vi "constroi_atp_bakcup.vi"() -> ()   [LabVIEW 2014]
uses:
  <vilib>/Utility/file.llb/Read From Spreadsheet File (DBL).vi
  <vilib>/Utility/file.llb/Read From Spreadsheet File (string).vi
panel:
  in  "Capacitors":string="  N0083A                      1.  .001  36.8                                   0\n  N0083B                      1.  .001  36.8                                   0\n  N0083C                      1.  .001  36.8                                   0\n  N0088A                      1.  .001   9.2                                   0\n  N0090B                      1.  .001   9.2                                   0\n  N0092C                      1.  .001   9.2                                   0"
  out "Switches":string
  out "chaves":dbl[][](array[numeric])
  out "Loads":string
  in  "Frequência (Hz)":dbl=50.0
  in  "Fonte (V)":dbl=4160.0
  out "subarray":dbl[][](array[numeric])
  out "nós":dbl[](array[numeric])
  out "all rows 2":dbl[][](array[numeric]) format="%0.3f"
  out "Linhas":string
  out "Reatances":dbl[][](array[numeric])
  out "Resistances":dbl[][](array[numeric])
  out "config":dbl[](array[numeric])
  out "Para":dbl[](array[numeric])
  out "De":dbl[](array[numeric])
  out "all rows":dbl[][](array[numeric]) format="%0.3f"
  out "Distance (miles)":dbl[](array[numeric])
  out "size(s)":i32[](array[numeric])
  in  "file path (use dialog)":path=path "C:/Users/Flavio/Documents/ATPdata/work/teste.atp"
  out "concatenated string":string
  # "A                B              C"
  # "A"
  # "B"
  # "C"
  # "R     +     X"
  # "R     +     X"
  # "R     +     X"
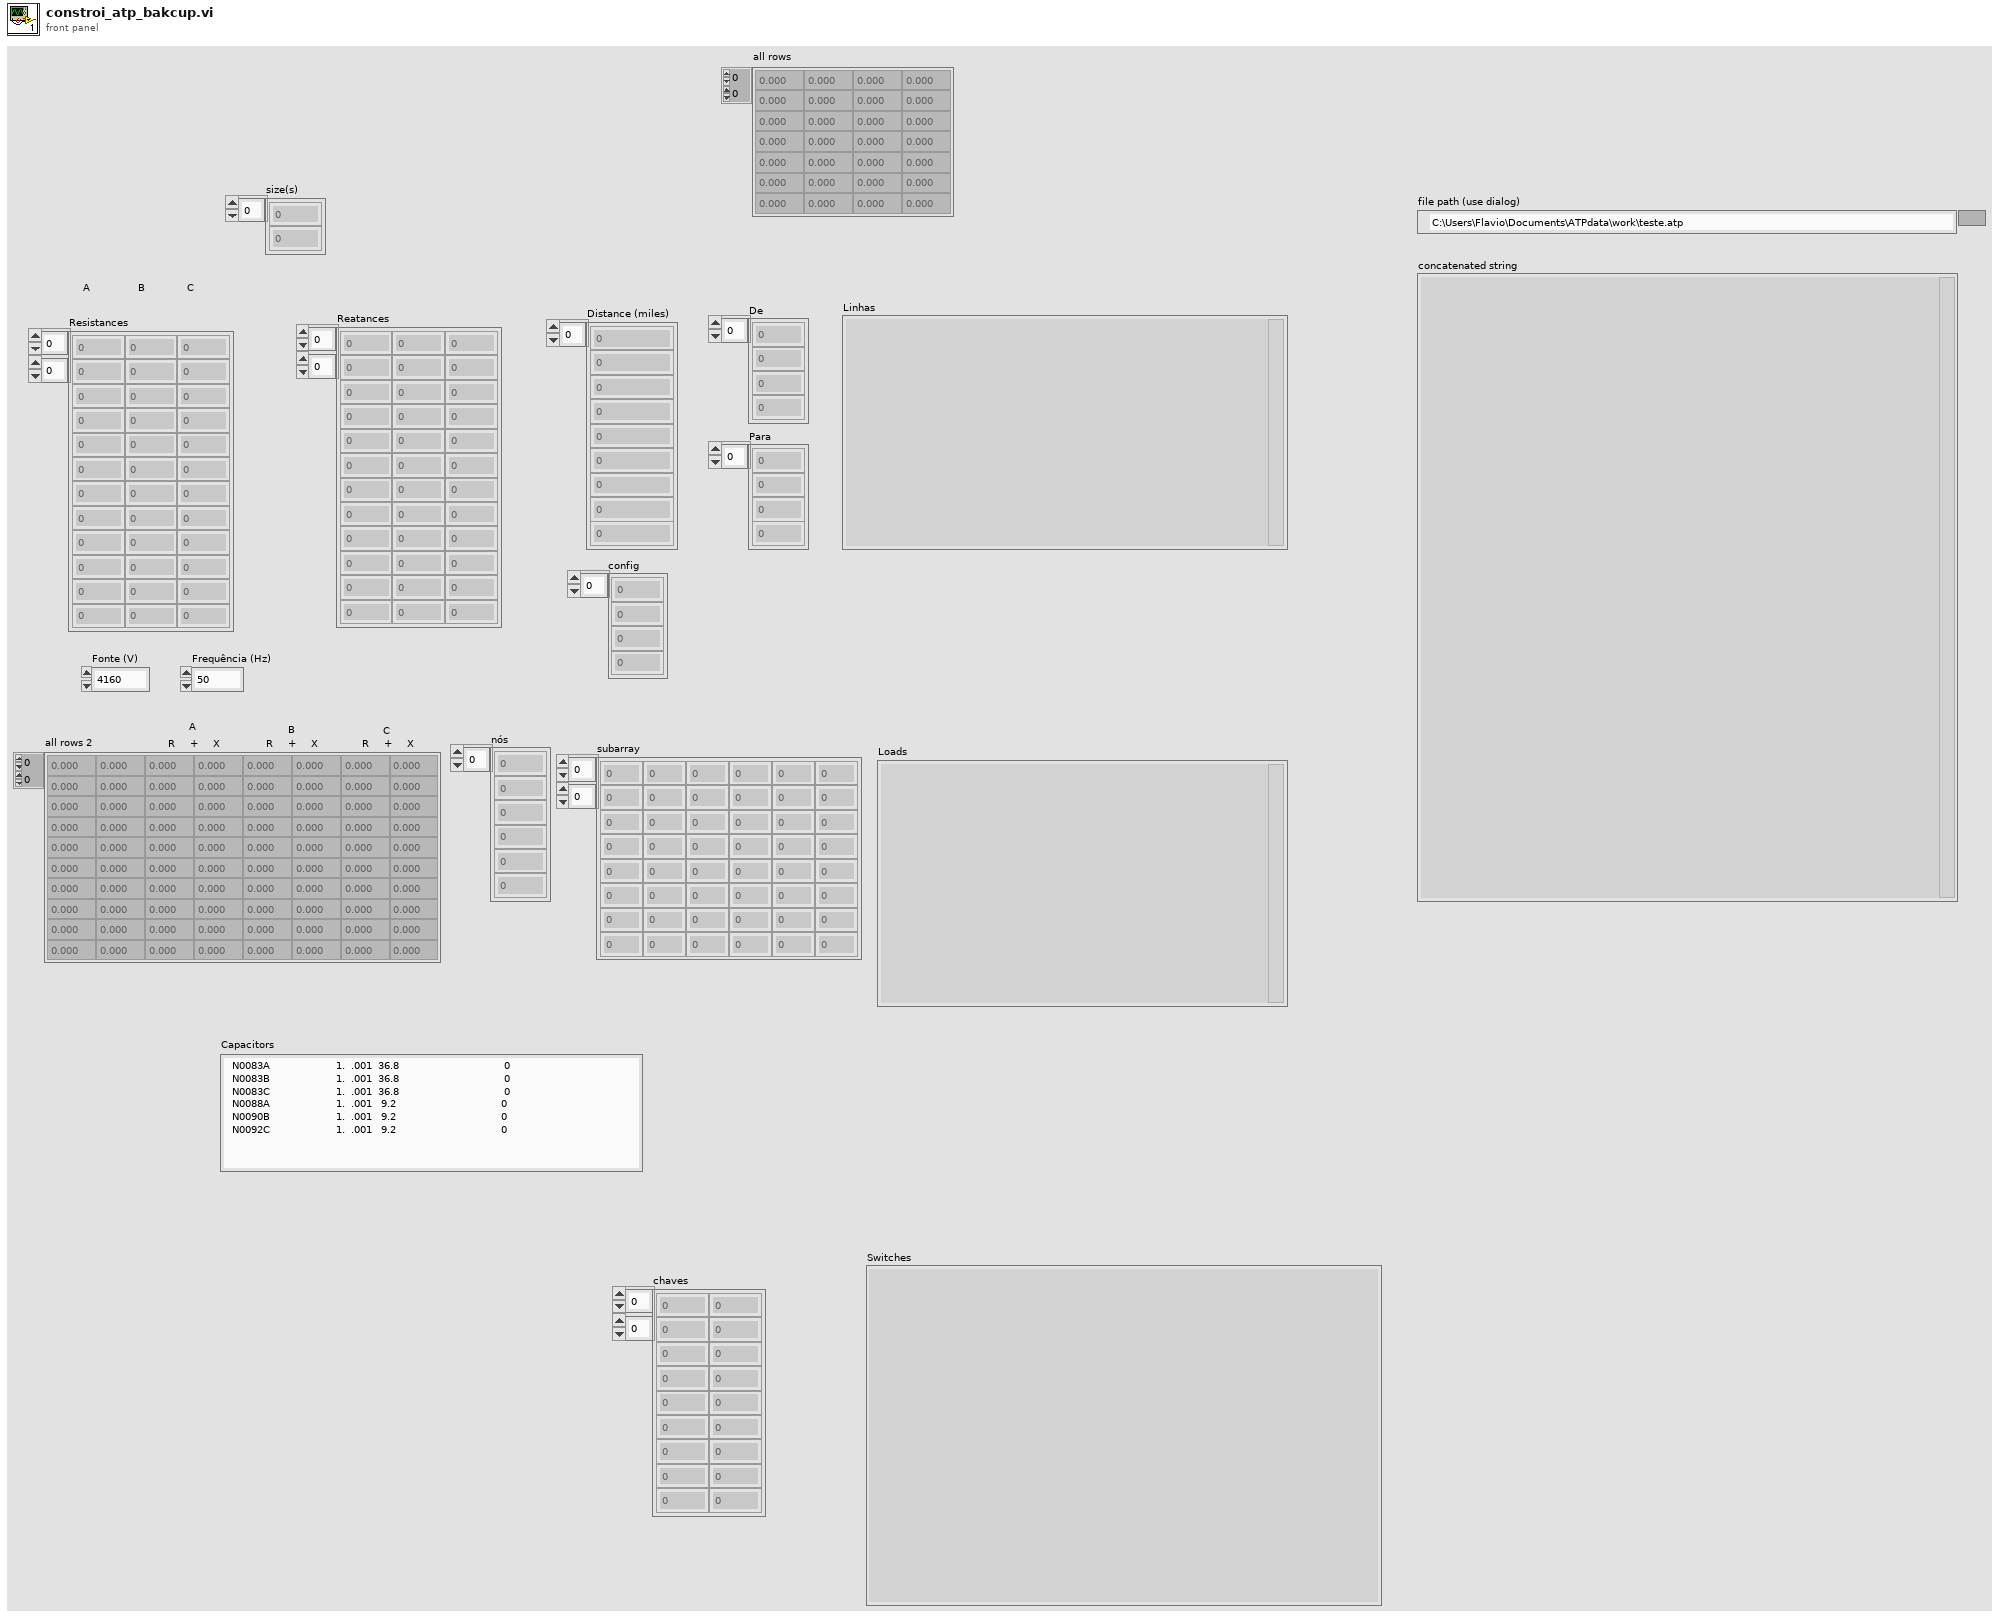
[diagram p1: front panel]
types:
  T1 = enum16{"open", "replace", "create", "open or create", "replace or create", "replace or create with confirmation"}
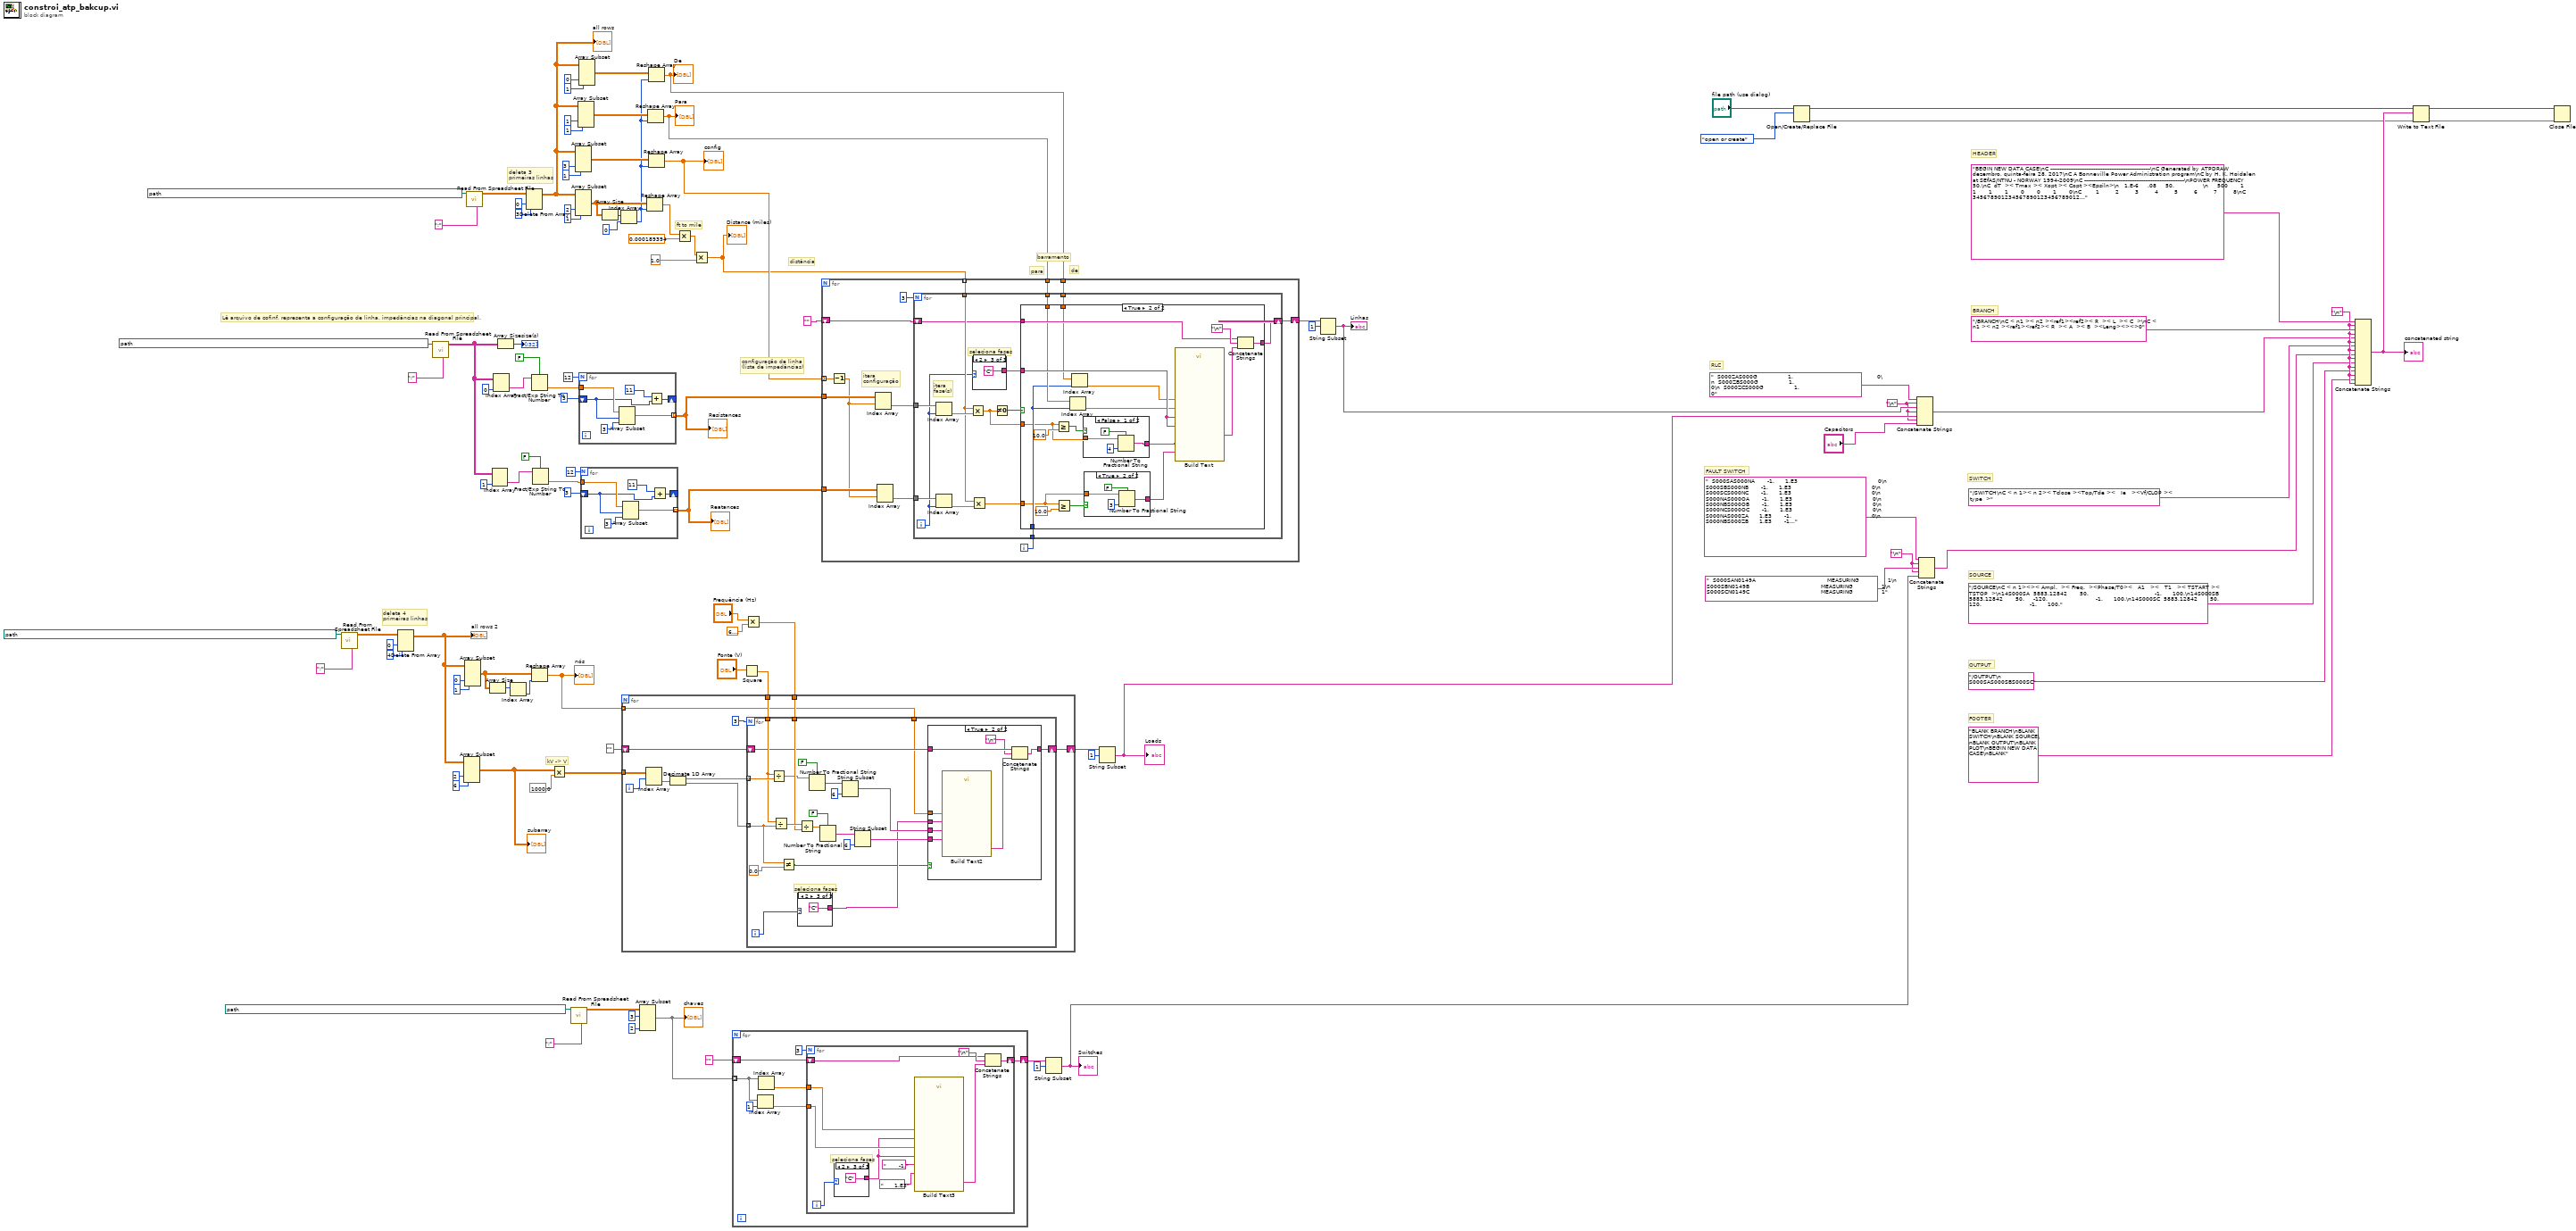
[diagram p0: block diagram]
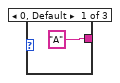
[diagram p2: hidden frame]
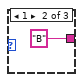
[diagram p3: hidden frame]
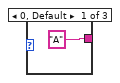
[diagram p5: hidden frame]
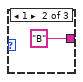
[diagram p6: hidden frame]
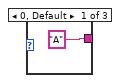
[diagram p7: hidden frame]
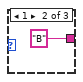
[diagram p8: hidden frame]
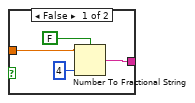
[diagram p10: hidden frame]
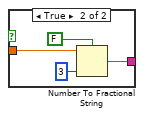
[diagram p11: hidden frame]
diagram:
  w2 = "\n"
  w5 = "\n"
  w107 = "\n"
  # "kV -> V"
  # "deleta 4\nprimeiras linhas"
  # "barramento"
  # "para"
  # "de"
  # "distância"
  # "configuração de linha \n(lista de impedâncias)"
  # "deleta 3\nprimeiras linhas"
  # "ft to mile"
  # "Lê arquivo de cofinf, representa a configuração de linha, impedâncias na diagonal principal."
  # "RLC"
  # "FAULT SWITCH"
  # "OUTPUT"
  # "FOOTER"
  # "SOURCE"
  # "SWITCH"
  # "BRANCH"
  # "HEADER"
  n1 = call-poly <vilib>:"Read From Spreadsheet File.vi"("delimiter (\\t)"=";" ("delimiter (\\t)"), "file path (dialog if empty)"=path "C:/Users/Flavio/Google Drive/Doutorado/Disciplinas/Mineração de Dados/Trabalho final/feeder123/spot loads data.csv") -> ("all rows"=w47:dbl[][])  [unwired: 5 in, 4 out]
  n2 = Delete From Array(array=w47, length=4, index (row)=0) -> (array with subset deleted=w38:dbl[][])  [unwired: 1 in, 1 out]
  "all rows 2" <- w38
  n3 = call-poly <vilib>:"Read From Spreadsheet File.vi"("delimiter (\\t)"=";" ("delimiter (\\t)"), "file path (dialog if empty)"=path "C:/Users/Flavio/Google Drive/Doutorado/Disciplinas/Mineração de Dados/Trabalho final/feeder123/config.csv") -> ("all rows"=w65:string[][])  [unwired: 5 in, 4 out]
  n4 = Array Subset(array=w38, index (col)=2 ("index"), length (col)=6 ("length")) -> (w32:dbl[][])  [unwired: 2 in]
  "subarray" <- w32
  n5 = Array Subset(array=w38, index (col)=0 ("index"), length (col)=1 ("length")) -> (w44:dbl[][])  [unwired: 2 in]
  n6 = call-poly <vilib>:"Read From Spreadsheet File.vi"("delimiter (\\t)"=";" ("delimiter (\\t)"), "file path (dialog if empty)"=path "C:/Users/Flavio/Google Drive/Doutorado/Disciplinas/Mineração de Dados/Trabalho final/feeder123/line data.csv") -> ("all rows"=w92:dbl[][])  [unwired: 5 in, 4 out]
  n7 = Array Size(array=w44) -> (size(s)=w43:i32[])
  n8 = Index Array(array=w65, index (col)=1 ("disabled index (col)")) -> (element=w59:string[])  [unwired: 1 in]
  n9 = Index Array(array=w65, index (col)=0 ("disabled index (col)")) -> (element=w63:string[])  [unwired: 1 in]
  n10 = Array Size(array=w65) -> (size(s)=→"size(s)":i32[])
  n11 = Index Array(array=w43) -> (element=w42:i32)  [unwired: 1 in]
  n12 = Delete From Array(array=w92, length=3, index (row)=0) -> (array with subset deleted=w74:dbl[][])  [unwired: 1 in, 1 out]
  "all rows" <- w74
  n13 = Reshape Array(w44, w42) -> (w41:dbl[])
  "nós" <- w41
  n14 = Fract/Exp String To Number(use system decimal point (T)=FALSE, string=w63) -> (number=w61:dbl[])  [unwired: 2 in, 1 out]
  n15 = Fract/Exp String To Number(use system decimal point (T)=FALSE, string=w59) -> (number=w60:dbl[])  [unwired: 2 in, 1 out]
  n16 = Multiply(x=w32, y=1000.0) -> (x*y=w30:dbl[][])
  n17 = call-poly <vilib>:"Read From Spreadsheet File.vi"("delimiter (\\t)"=";" ("delimiter (\\t)"), "file path (dialog if empty)"=path "C:/Users/Flavio/Google Drive/Doutorado/Disciplinas/Mineração de Dados/Trabalho final/feeder123/switch data modif.csv") -> ("all rows"=w22:dbl[][])  [unwired: 5 in, 4 out]
  n18 = Array Subset(array=w74, index (col)=3 ("index"), length (col)=1 ("length")) -> (w73:dbl[][])  [unwired: 2 in]
  n19 = Array Subset(array=w74, index (col)=2 ("index"), length (col)=1 ("length")) -> (w87:dbl[][])  [unwired: 2 in]
  n20 = Array Subset(array=w74, index (col)=1 ("index"), length (col)=1 ("length")) -> (w71:dbl[][])  [unwired: 2 in]
  n21 = Array Subset(array=w74, index (col)=0 ("index"), length (col)=1 ("length")) -> (w72:dbl[][])  [unwired: 2 in]
  n22 = for {
    N: 12 -> [_]
    tunnel: w61 -> [w115]
    shift-right: [w111] -> _
    shift-left: 3 ("length") -> [w112]
    tunnel: [w110] -> w69 mode=indexing
    n23 = Array Subset(array=w115, index=w112, length=3) -> (w110:dbl[])
    n24 = Add(x=11 ("length"), y=w112) -> (x+y=w111:i32)
  }
  "Resistances" <- w69
  n25 = for {
    N: 12 -> [_]
    tunnel: w60 -> [w121]
    shift-right: [w117] -> _
    shift-left: 3 ("length") -> [w118]
    tunnel: [w116] -> w57 mode=indexing
    n26 = Array Subset(array=w121, index=w118, length=3) -> (w116:dbl[])
    n27 = Add(x=11 ("length"), y=w118) -> (x+y=w117:i32)
  }
  "Reatances" <- w57
  n28 = Array Size(array=w87) -> (size(s)=w86:i32[])
  n29 = Index Array(array=w86, index=0) -> (element=w70:i32)
  n30 = Array Subset(array=w22, index (row)=3 ("index"), length (col)=2 ("length")) -> (w19:dbl[][])  [unwired: 2 in]
  "chaves" <- w19
  n31 = Reshape Array(w87, w70) -> (w84:dbl[])
  n32 = Reshape Array(w71, w70) -> (w55:dbl[])
  "Para" <- w55
  n33 = Reshape Array(w73, w70) -> (w64:dbl[])
  "config" <- w64
  n34 = Reshape Array(w72, w70) -> (w54:dbl[])
  "De" <- w54
  n35 = Multiply(x=w84, y=0.000189394) -> (x*y=w53:dbl[])
  n36 = Multiply(x=w53, y=1.0) -> (x*y=w52:dbl[])
  "Distance (miles)" <- w52
  n37 = for {
    tunnel: w19 -> [w128] mode=indexing
    shift-right: [w125] -> w16
    shift-left: "" -> [w126]
    n38 = Index Array(array=w128, index=1) -> (element=w123:dbl)
    n39 = Index Array(array=w128) -> (element=w124:dbl)  [unwired: 1 in]
    n40 = for {
      N: 3 -> [_]
      shift-right: [w138] -> w125
      shift-left: w126 -> [w129]
      tunnel: w124 -> [w137]
      tunnel: w123 -> [w136]
      i -> [w135]
      # "seleciona fases"
      n41 = case shown="2" w135 {
        tunnel: ["A" "B" "C"] -> w134
        frame 0, Default {
        }
        frame 1 {
        }
        frame 2 {
        }
      }
      n42 = call "Build Text3"("fase_out"=w134, "Topen"="      1.E3", "de"=w137, "fase_in"=w134, "para"=w136, "Tclose"="       -1.") -> ("Result"=w131:string)  [unwired: 8 in, 1 out]
      n43 = Concatenate Strings(w129, "\n", w131) -> (w138:string)
    }
  }
  n44 = Square(x="Fonte (V)") -> (x^2=w36:dbl)
  n45 = Multiply(x="Frequência (Hz)", y=6.283185307179586) -> (x*y=w33:dbl)
  n46 = for {
    tunnel: w41 -> [w144] mode=indexing
    tunnel: w30 -> [w152]
    tunnel: w36 -> [w146]
    tunnel: w33 -> [w145]
    shift-right: [w142] -> w28
    shift-left: "" -> [w143]
    i -> [w151]
    n47 = Index Array(array=w152, index (row)=w151) -> (element=w149:dbl[])  [unwired: 1 in]
    n48 = Decimate 1D Array(w149) -> (w148:dbl[], w147:dbl[])
    n49 = for {
      N: 3 -> [_]
      tunnel: w148 -> [w174] mode=indexing
      tunnel: w147 -> [w163] mode=indexing
      tunnel: w146 -> [w173]
      tunnel: w145 -> [w171]
      tunnel: w144 -> [w157]
      shift-right: [w161] -> w142
      shift-left: w143 -> [w162]
      i -> [w164]
      # "seleciona fases"
      n50 = Divide(x=w173, y=w174) -> (x/y=w170:dbl)
      n51 = Divide(x=w173, y=w163) -> (x/y=w172:dbl)
      n52 = Not Equal?(x=w163, y=0.0 ("x")) -> (x != y?=w156:bool)
      n53 = case shown="2" w164 {
        tunnel: ["A" "B" "C"] -> w158
        frame 0, Default {
        }
        frame 1 {
        }
        frame 2 {
        }
      }
      n54 = Divide(x=w172, y=w171) -> (x/y=w169:dbl)
      n55 = Number To Fractional String(use system decimal point (T)=FALSE, number=w170) -> (F-format string=w168:string)  [unwired: 2 in]
      n56 = Number To Fractional String(use system decimal point (T)=FALSE, number=w169) -> (F-format string=w166:string)  [unwired: 2 in]
      n57 = String Subset(string=w168, length (rest)=6 ("length (rest)")) -> (substring=w159:string)  [unwired: 1 in]
      n58 = String Subset(string=w166, length (rest)=6 ("length (rest)")) -> (substring=w160:string)  [unwired: 1 in]
      n59 = case shown="True" w156 {
        tunnel: w162 -> [w175 w183]
        tunnel: [w175 w180] -> w161
        tunnel: w160 -> [_ w179]
        tunnel: w159 -> [_ w178]
        tunnel: w158 -> [_ w177]
        tunnel: w157 -> [_ w176]
        frame False {
        }
        frame True {
          n60 = call "Build Text2"("reatancia"=w179, "no"=w176, "fase"=w177, "resistencia"=w178) -> ("Result"=w181:string)  [unwired: 10 in, 1 out]
          n61 = Concatenate Strings(w183, "\n", w181) -> (w180:string)
        }
      }
    }
  }
  n62 = for {
    tunnel: w69 -> [w199]
    tunnel: w57 -> [w196]
    tunnel: w64 -> [w188] mode=indexing
    tunnel: w52 -> [w194] mode=indexing
    shift-right: [w192] -> w25
    shift-left: "" -> [w193]
    tunnel: w55 -> [w191]
    tunnel: w54 -> [w190]
    i -> [w189]
    # "itera\nconfiguração"
    n63 = Decrement(x=w188) -> (x-1=w187:dbl)
    n64 = Index Array(array=w199, index (row)=w187) -> (element=w198:dbl[])  [unwired: 1 in]
    n65 = Index Array(array=w196, index (row)=w187) -> (element=w197:dbl[])  [unwired: 1 in]
    n66 = for {
      N: 3 -> [_]
      tunnel: w198 -> [w214]
      tunnel: w197 -> [w213]
      tunnel: w194 -> [w210]
      shift-right: [w207] -> w192
      shift-left: w193 -> [w208]
      tunnel: w191 -> [w202]
      tunnel: w190 -> [w201]
      tunnel: w189 -> [w200]
      i -> [w206]
      # "seleciona fases"
      # "itera\nfase(s)"
      n67 = Index Array(array=w214, index=w206) -> (element=w212:dbl)
      n68 = Index Array(array=w213, index=w206) -> (element=w211:dbl)
      n69 = Multiply(x=w210, y=w212) -> (x*y=w204:dbl)
      n70 = Multiply(x=w210, y=w211) -> (x*y=w205:dbl)
      n71 = case shown="2" w206 {
        tunnel: ["A" "B" "C"] -> w203
        frame 0, Default {
        }
        frame 1 {
        }
        frame 2 {
        }
      }
      n72 = Not Equal To 0?(x=w204) -> (x != 0?=w209:bool)
      n73 = case shown="True" w209 {
        tunnel: w208 -> [w218 w234]
        tunnel: [w218 w235] -> w207
        tunnel: w205 -> [_ w221]
        tunnel: w204 -> [_ w223]
        tunnel: w203 -> [_ w232]
        tunnel: w202 -> [_ w231]
        tunnel: w201 -> [_ w230]
        tunnel: w200 -> [_ w227]
        frame False {
        }
        frame True {
          n74 = Greater Or Equal?(x=w223, y=10.0) -> (x >= y?=w226:bool)
          n75 = Greater Or Equal?(x=w221, y=10.0) -> (x >= y?=w220:bool)
          n76 = Index Array(array=w231, index=w227) -> (element=w229:dbl)
          n77 = Index Array(array=w230, index=w227) -> (element=w228:dbl)
          n78 = case shown="False" w226 {
            tunnel: w223 -> [w247 w251]
            tunnel: [w246 w250] -> w222
            frame False {
              n79 = Number To Fractional String(use system decimal point (T)=FALSE, number=w247, precision (6)=i16 4) -> (F-format string=w246:string)  [unwired: 1 in]
            }
            frame True {
              n80 = Number To Fractional String(use system decimal point (T)=FALSE, number=w251, precision (6)=i16 3) -> (F-format string=w250:string)  [unwired: 1 in]
            }
          }
          n81 = case shown="True" w220 {
            tunnel: w221 -> [w239 w243]
            tunnel: [w238 w242] -> w219
            frame False {
              n82 = Number To Fractional String(use system decimal point (T)=FALSE, number=w239, precision (6)=i16 4) -> (F-format string=w238:string)  [unwired: 1 in]
            }
            frame True {
              n83 = Number To Fractional String(use system decimal point (T)=FALSE, number=w243, precision (6)=i16 3) -> (F-format string=w242:string)  [unwired: 1 in]
            }
          }
          n84 = call "Build Text"("fase_out"=w232, "reatancia"=w219, "de"=w228, "fase_in"=w232, "para"=w229, "resistencia"=w222) -> ("Result"=w233:string)  [unwired: 8 in, 1 out]
          n85 = Concatenate Strings(w234, "\n", w233) -> (w235:string)
        }
      }
    }
  }
  n86 = String Subset(string=w16, offset (0)=1) -> (substring=w15:string)  [unwired: 1 in]
  "Switches" <- w15
  n87 = String Subset(string=w28, offset (0)=1) -> (substring=w13:string)  [unwired: 1 in]
  "Loads" <- w13
  n88 = String Subset(string=w25, offset (0)=1) -> (substring=w12:string)  [unwired: 1 in]
  "Linhas" <- w12
  n89 = Open/Create/Replace File(file path (use dialog)="file path (use dialog)", operation (0:open)=T1."open or create") -> (refnum out=w101:refnum<file>, error out=w102:errorcluster)  [unwired: 4 in, 1 out]
  n90 = Concatenate Strings("  S000ZAS000G                 1.                                               0\n  S000ZBS000G                 1.                                               0\n  S000ZCS000G                 1.                                               0", w2, w12, w2, w13, w2, "Capacitors") -> (w14:string)
  n91 = Concatenate Strings("  S000SAS000NA       -1.      1.E3                                             0\n  S000SBS000NB       -1.      1.E3                                             0\n  S000SCS000NC       -1.      1.E3                                             0\n  S000NAS000OA       -1.      1.E3                                             0\n  S000NBS000OB       -1.      1.E3                                             0\n  S000NCS000OC       -1.      1.E3                                             0\n  S000NAS000ZA      1.E3       -1.                                             0\n  S000NBS000ZB      1.E3       -1.                                             0\n  S000NCS000ZC      1.E3       -1.                                             0\n  S000G             1.E3       -1.                                             0", w5, "  S000SAN0149A                                        MEASURING                1\n  S000SBN0149B                                        MEASURING                1\n  S000SCN0149C                                        MEASURING                1", w5, w15) -> (w8:string)
  n92 = Concatenate Strings("BEGIN NEW DATA CASE\nC --------------------------------------------------------\nC Generated by ATPDRAW  dezembro, quinta-feira 28, 2017\nC A Bonneville Power Administration program\nC by H. K. Høidalen at SEfAS/NTNU - NORWAY 1994-2009\nC --------------------------------------------------------\nPOWER FREQUENCY                      50.\nC  dT  >< Tmax >< Xopt >< Copt ><Epsiln>\n   1.E-6     .08     50.                \n     500       1       1       1       1       0       0       1       0\nC        1         2         3         4         5         6         7         8\nC 345678901234567890123456789012345678901234567890123456789012345678901234567890", w107, "/BRANCH\nC < n1 >< n2 ><ref1><ref2>< R  >< L  >< C  >\nC < n1 >< n2 ><ref1><ref2>< R  >< A  >< B  ><Leng><><>0", w107, w14, w107, "/SWITCH\nC < n 1>< n 2>< Tclose ><Top/Tde ><   Ie   ><Vf/CLOP ><  type  >", w107, w8, w107, "/SOURCE\nC < n 1><>< Ampl.  >< Freq.  ><Phase/T0><   A1   ><   T1   >< TSTART >< TSTOP  >\n14S000SA  5883.12842       50.                                     -1.      100.\n14S000SB  5883.12842       50.     -120.                           -1.      100.\n14S000SC  5883.12842       50.      120.                           -1.      100.", w107, "/OUTPUT\n  S000SAS000SBS000SC", w107, "BLANK BRANCH\nBLANK SWITCH\nBLANK SOURCE\nBLANK OUTPUT\nBLANK PLOT\nBEGIN NEW DATA CASE\nBLANK", w107) -> (w105:string)
  "concatenated string" <- w105
  n93 = Write to Text File(file (use dialog)=w101, text=w105, error in=w102) -> (refnum out=w104:refnum<file>, error out=w103:errorcluster)  [unwired: 1 in, 1 out]
  n94 = Close File(refnum=w104, error in=w103) -> ()  [unwired: 2 out]
